vi "Exercise2Part1BTS.vi"() -> ()   [LabVIEW 2014]
panel:
  in  "stop":bool
  out "B":dbl
  out "A":dbl
  out "A+B":dbl
  # "+"
  # "="
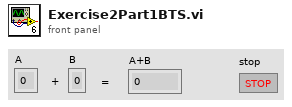
[diagram p1: front panel]
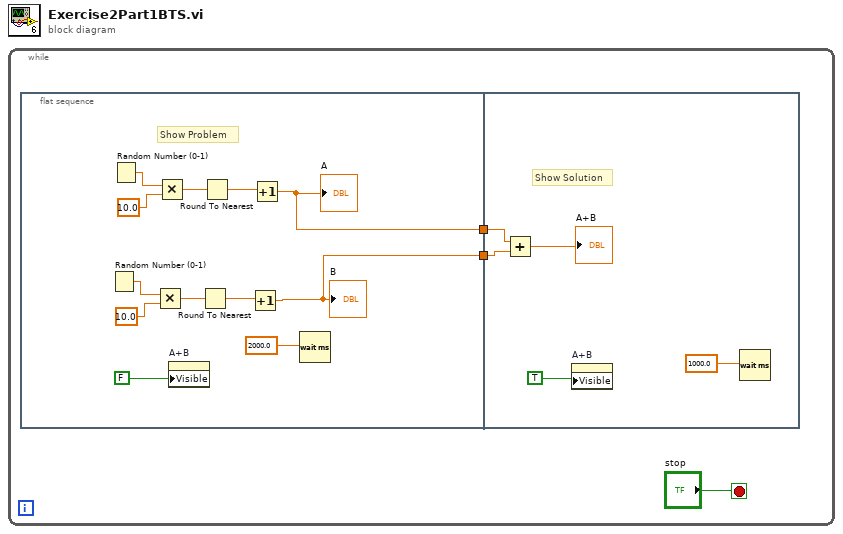
[diagram p0: block diagram]
diagram:
  n1 = while {
    stop <- "stop" stop-if-true
    n2 = flat-sequence {
      tunnel: [w5] -> w2
      tunnel: [w4] -> w1
      tunnel: w2 -> [w16]
      tunnel: w1 -> [w17]
      frame #0 {
        # "Show Problem"
        n3 = Random Number (0-1)() -> (number: 0 to 1=w10:dbl)
        n4 = Random Number (0-1)() -> (number: 0 to 1=w6:dbl)
        n5 = Multiply(x=w10, y=10.0) -> (x*y=w12:dbl)
        n6 = Multiply(x=w6, y=10.0) -> (x*y=w8:dbl)
        n7 = property on="A+B" class="DigNum (strict)"("Visible"=FALSE) -> ()  [unwired: 2 in, 2 out]
        n8 = Round To Nearest(number=w12) -> (nearest integer value=w13:dbl)
        n9 = Round To Nearest(number=w8) -> (nearest integer value=w9:dbl)
        n10 = Increment(x=w13) -> (x+1=w4:dbl)
        "B" <- w4
        n11 = Increment(x=w9) -> (x+1=w5:dbl)
        "A" <- w5
        n12 = Wait (ms)(milliseconds to wait=2000.0) -> ()  [unwired: 1 out]
      }
      frame #1 {
        # "Show Solution"
        n13 = Add(x=w16, y=w17) -> (x+y=→"A+B":dbl)
        n14 = property on="A+B" class="DigNum (strict)"("Visible"=TRUE) -> ()  [unwired: 2 in, 2 out]
        n15 = Wait (ms)(milliseconds to wait=1000.0) -> ()  [unwired: 1 out]
      }
    }
  }
